vi "Gyroscope.vi"(8 "error in (no error)":errorcluster, 9 "Reset YAW":bool, 11 "IMU in":refnum<class "IMU.lvclass">) -> (0 "error out":errorcluster, 1 "YAW (rad)":dbl, 2 "YAW (degree)":dbl, 3 "IMU out":refnum<class "IMU.lvclass">, 5 "IMU":dbl[](array[numeric]))   [LabVIEW 2020]
uses:
  <vilib>/High Genius/HG_WSI_Tookit/Dependencies/Library/IMU/IMU.lvclass
  C:/Program Files (x86)/National Instruments/LabVIEW 2020/vi.lib/High Genius/HG_WSI_Tookit/Dependencies/Library/HG_LIB/HG_LIB.lvclass
  <vilib>/High Genius/HG_WSI_Tookit/Dependencies/Library/HG_LIB/HG_LIB.lvclass
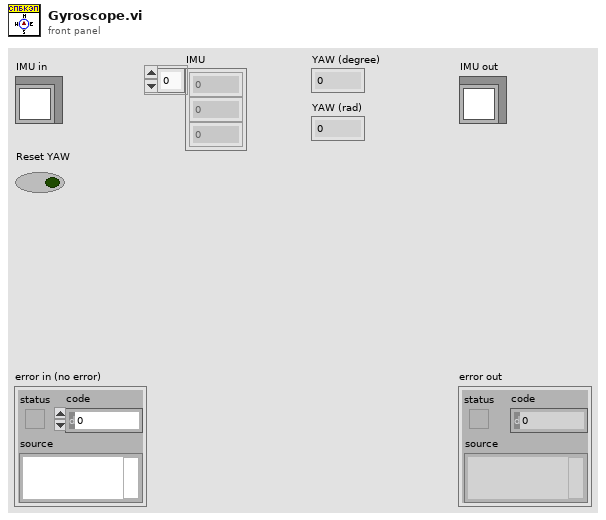
[diagram p1: front panel]
types:
  T1 = cluster{"data":cluster{"ai22":sgl, "ai23":sgl, "ai24":sgl, "ai25":sgl, "pulse12":i32, "pulse13":i32, "pwm14":i32, "pwm15":i32, "pwm16":i32, "do17":bool, "do18":bool, "do19":bool, "do20":bool, "do21":bool, "di11":bool, "di9":bool, "motor0":u8, "motor1":u8, "motor2":u8, "motor3":u8, "dir00":u8, "dir01":u8, "dir02":u8, "dir03":u8, "dir10":u8, "dir11":u8, "dir12":u8, "dir13":u8, "limit0":bool, "limit1":bool, "limit2":bool, "limit3":bool, "limit4":bool, "limit5":bool, "limit6":bool, "limit7":bool, "lsb0H":u8, "lsb1H":u8, "lsb2H":u8, "lsb3H":u8, "lsb0L":u8, "lsb1L":u8, "lsb2L":u8, "lsb3L":u8, "enc0_counters":u32, "enc1_counters":u32, "enc2_counters":u32, "enc3_counters":u32, "counter10":u32, "counter8":u32, "reset_enc0":bool, "reset_enc1":bool, "reset_enc2":bool, "reset_enc3":bool, "pitch":sgl, "roll":sgl, "yaw":sgl, "zero_yaw":bool}}
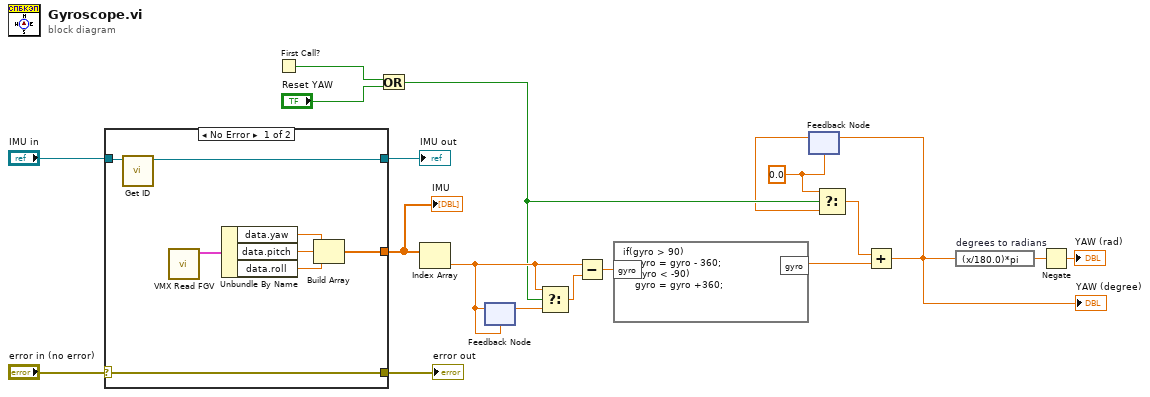
[diagram p0: block diagram]
diagram:
  w4 = 0.0
  n1 = case shown="No Error" "error in (no error)" {
    selector: "error in (no error)" -> [w24 w29]
    tunnel: [w24 w29] -> w9
    tunnel: [w27 w28] -> w17
    tunnel: "IMU in" -> [w26 w28]
    tunnel: [w20 _] -> w12
    frame No Error {
      n2 = call <vilib>:"Get ID.vi"("HG_LIB in"=w26) -> ("HG_LIB out"=w27:refnum<class "IMU.lvclass">)  [unwired: 9 in, 1 out]
      n3 = call <vilib>:"VMX Read FGV.vi"() -> ("Read Data"=w25:T1)  [unwired: 10 in, 1 out]
      n4 = Unbundle By Name(w25) -> ("data.yaw"=w23:sgl, "data.pitch"=w22:sgl, "data.roll"=w21:sgl)
      n5 = Build Array(w23, w22, w21) -> (w20:sgl[])
    }
    frame Error {
    }
  }
  "error out" <- w9
  "IMU out" <- w17
  "IMU" <- w12
  n6 = First Call?() -> (First Call?: T/F=w11:bool)
  n7 = Or(x=w11, y="Reset YAW") -> (x .or. y?=w3:bool)
  n8 = Index Array(array=w12) -> (element=w5:sgl)  [unwired: 1 in]
  n9 = feedback #1(w5) -> (w15:sgl)
  n10 = feedback-in #1(w5) -> ()
  n11 = Select(t=w5, s=w3, f=w15) -> (s? t:f=w14:sgl)
  n12 = Subtract(x=w5, y=w14) -> (x-y=w16:sgl)
  n13 = formula code="if(gyro > 90)\n    gyro = gyro - 360;\n if(gyro < -90)\n    gyro = gyro +360;"("gyro"=w16) -> ("gyro"=w6:sgl)
  n14 = feedback #2(w4) -> (w2:dbl)
  n15 = Select(t=w4, s=w3, f=w2) -> (s? t:f=w13:dbl)
  n16 = Add(x=w13, y=w6) -> (x+y=w1:dbl)
  "YAW (degree)" <- w1
  n17 = feedback-in #2(w1) -> ()
  n18 = expression code="(x/180.0)*pi" "degrees to radians"(w1) -> (w8:dbl)
  n19 = Negate(x=w8) -> (-x=→"YAW (rad)":dbl)
